vi "Requests.vi"(8 "error in (no error)":errorcluster, 9 "write enable":bool=TRUE, 11 "ICPCON ET in":refnum<class "ICPCON ET-7042.lvclass">) -> (0 "error out":errorcluster, 3 "ICPCON ET out":refnum<class "ICPCON ET-7042.lvclass">)   [LabVIEW 2021, in "ICPCON ET-7042.lvclass"]
uses:
  ICPCON ET-7042.lvclass
  D:/my_projects/projects/Algorithms/Labview/21/Modbus/MB_TCP2/MB_TCP.lvclass
  MB_TCP.lvclass/MB_TCP.ctl
  NI_modbus_upd/Ctl/Unit_ID.ctl
  NI_modbus_upd/TCP/TCP.lvclass/TCP.ctl
  NI_modbus_upd/Master Function Definition/Responses/Read Coils Response.vi
  NI_modbus_upd/Master Function Definition/Requests/Read Coils Request.vi
  NI_modbus_upd/Master network read write.vi
  NI_modbus_upd/Function data mismatch error1.vi
  NI_modbus_upd/Master Function Definition/Responses/Write Multiple Coils Response.vi
  NI_modbus_upd/Master Function Definition/Requests/Write Multiple Coils Request.vi
  NI_modbus_upd/Utility/Bytes to Bits1.vi
  NI_modbus_upd/Error Generator1.vi
  NI_modbus_upd/Function code mismatch error1.vi
  NI_modbus_upd/Modbus Data Unit (PDU)/Construct PDU1.vi
  NI_modbus_upd/Read ADU Packet Master.vi
  NI_modbus_upd/Write ADU Packet Master.vi
  NI_modbus_upd/Utility/Bits to Bytes1.vi
  NI_modbus_upd/Modbus Data Unit (PDU)/Unflatten to PDU1.vi
  NI_modbus_upd/TCP/Protocol Read.vi
  NI_modbus_upd/TCP/Protocol Write.vi
  <vilib>/Utility/error.llb/Clear Errors.vi
  NI_modbus_upd/Modbus Data Unit (PDU)/Deconstruct PDU1.vi
  NI_modbus_upd/TCP/TCP.lvclass
  ICPCON Registers/ICPCON Registers.lvlib
  MB_TCP.lvclass
  NI_modbus_upd/NI_modbus_upd.lvlib
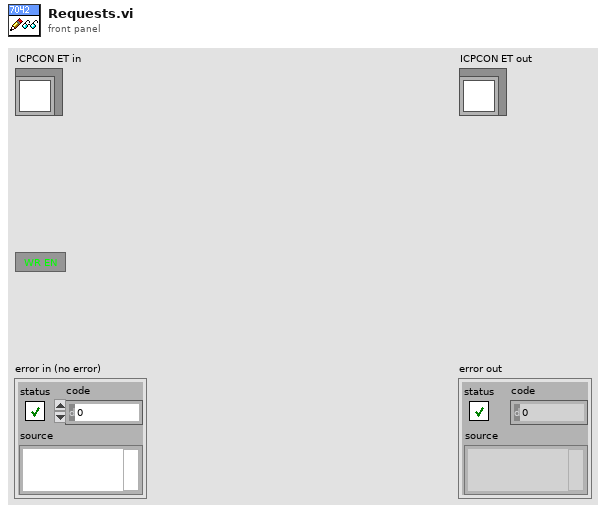
[diagram p1: front panel]
types:
  T1 = typedef "NI_modbus_upd.lvlib/Unit_ID.ctl" = cluster{"Protocol ID":u16, "Unit ID":u8}
  T2 = typedef "ICPCON Registers.lvlib/ICPCON Data.ctl" = cluster{"UTF":refnum<data-value>, "DI":refnum<data-value>, "DW":refnum<data-value>, "DO":refnum<data-value>, "IR":refnum<data-value>, "WR":refnum<data-value>, "OR":refnum<data-value>, "modified":refnum<data-value>}
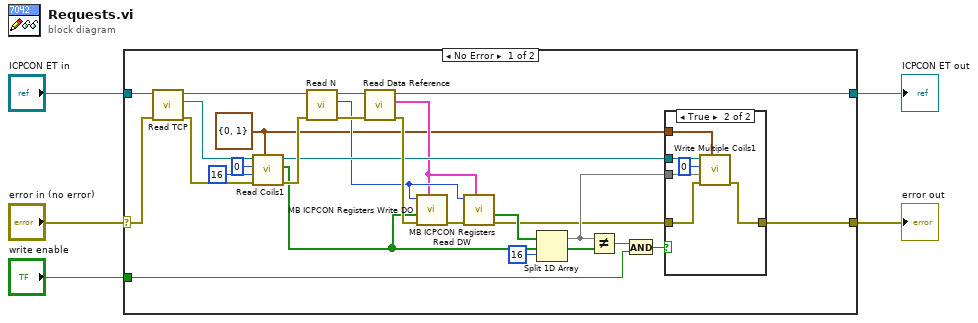
[diagram p0: block diagram]
diagram:
  n1 = case shown="No Error" "error in (no error)" {
    selector: "error in (no error)" -> [w22 w40]
    tunnel: [w12 w40] -> w3
    tunnel: [w27 w39] -> w4
    tunnel: "ICPCON ET in" -> [w29 w39]
    tunnel: "write enable" -> [w7 _]
    frame No Error {
      w6 = T1 {"Protocol ID"=0, "Unit ID"=1} ("Unit_ID")
      n2 = call "Read TCP.vi"("error in (no error)"=w22, "MB_TCP in"=w29) -> ("error out"=w23:errorcluster, "TCP"=w26:refnum<class "TCP.lvclass">, "MB_TCP out"=w28:refnum<class "ICPCON ET-7042.lvclass">)  [unwired: 7 in]
      n3 = call "Read Coils1.vi"("Unit_ID"=w6, "error in (no error)"=w23, "number of coils"=u16 16, "starting address"=u16 0, "Modbus master in"=w26) -> ("error out"=w21:errorcluster, "coil values"=w8:bool[], "Modbus master out"=w11:refnum<class "TCP.lvclass">)  [unwired: 4 in]
      n4 = call "Read N.vi"("error in (no error)"=w21, "MB_TCP in"=w28) -> ("error out"=w31:errorcluster, "N"=w10:i32, "MB_TCP out"=w30:refnum<class "ICPCON ET-7042.lvclass">)  [unwired: 7 in]
      n5 = call "Read Data Reference.vi"("error in (no error)"=w31, "MB_TCP in"=w30) -> ("error out"=w20:errorcluster, "Data"=w9:T2, "MB_TCP out"=w27:refnum<class "ICPCON ET-7042.lvclass">)  [unwired: 7 in]
      n6 = call "MB ICPCON Registers Write DO.vi"("Data Reference"=w9, "error in (no error)"=w20, "Bits In"=w8, "N"=w10) -> ("error out"=w13:errorcluster)  [unwired: 7 in]
      n7 = call "MB ICPCON Registers Read DW.vi"("Data Reference"=w9, "error in (no error)"=w13, "N"=w10) -> ("error out"=w14:errorcluster, "Bits out"=w17:bool[])  [unwired: 7 in]
      n8 = Split 1D Array(array=w17, index=16 ("length")) -> (first subarray=w15:bool[])  [unwired: 1 out]
      n9 = Not Equal?(x=w15, y=w8) -> (x != y?=w19:bool)
      n10 = And(x=w19, y=w7) -> (x .and. y?=w18:bool)
      n11 = case shown="True" w18 {
        tunnel: w14 -> [w32 w35]
        tunnel: [w32 w33] -> w12
        tunnel: w15 -> [_ w36]
        tunnel: w11 -> [_ w38]
        tunnel: w6 -> [_ w37]
        frame False {
        }
        frame True {
          n12 = call "Write Multiple Coils1.vi"("Unit_ID"=w37, "error in (no error)"=w35, "coil values"=w36, "starting address"=u16 0, "Modbus master in"=w38) -> ("error out"=w33:errorcluster)  [unwired: 5 in, 1 out]
        }
      }
    }
    frame Error {
    }
  }
  "error out" <- w3
  "ICPCON ET out" <- w4
